vi "link url.vi"(0 "服务器信息":T1={"host"="121.36.219.111", "port"=8020, "user"="std", "password"="std23506"}, 1 "远端地址":string="/updatefiles/OneStation/V4/版本升级文档.txt") -> (14 "url":string, 15 "file name":string)   [LabVIEW 2016, in "数据传输系统-04.lvlib" / "update.lvlib"]
uses:
  update.lvlib
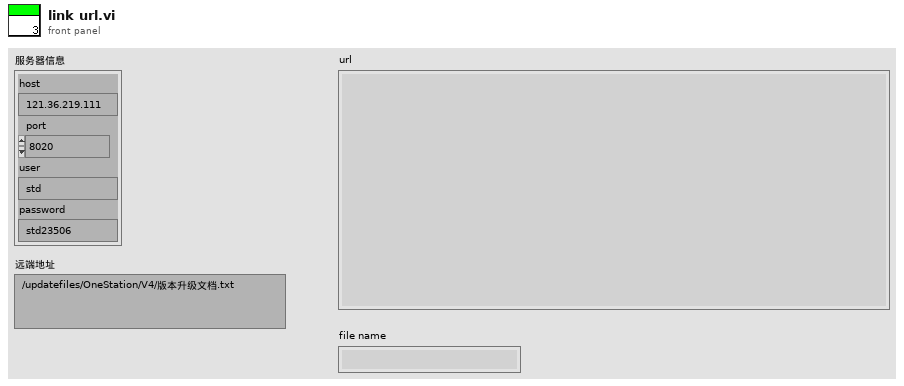
[diagram p1: front panel]
types:
  T1 = cluster{"host":string, "port":u16, "user":string, "password":string}
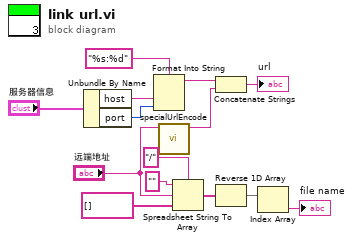
[diagram p0: block diagram]
diagram:
  n1 = Unbundle By Name("服务器信息") -> ("host"=w12:string, "port"=w11:u16)
  n2 = Format Into String(format string="%s:%d" ("格式字符串"), w12, w11) -> (resulting string=w10:string)  [unwired: 2 in, 1 out]
  n3 = call "specialUrlEncode.vi"("str"="远端地址") -> ("UrlEncode"=w9:string)  [unwired: 10 in]
  n4 = Spreadsheet String To Array(delimiter (Tab)="/", format string="" ("格式字符串"), spreadsheet string="远端地址", array type (2D Dbl)=string[] []) -> (array=w3:string[])
  n5 = Concatenate Strings(w10, w9) -> (→"url":string)
  n6 = Reverse 1D Array(array=w3) -> (reversed array=w2:string[])
  n7 = Index Array(array=w2) -> (element=→"file name":string)  [unwired: 1 in]
